vi "Compute Phasor Ratio References from UC Intersections.vi"(7 "mu+":dbl, 8 "error in (no error)":errorcluster, 9 "mu-":dbl, 10 "Phasor 1 (g, s)":T1, 11 "Phasor 2 (g, s)":T1) -> (0 "error out":errorcluster, 2 "Reference Phasor 2 (g, s)":T1, 3 "Reference Phasor 1 (g, s)":T1)   [LabVIEW 2021, in "Phasor.lvlib"]
uses:
  Phasor (g, s).ctl
  Phasor.lvlib
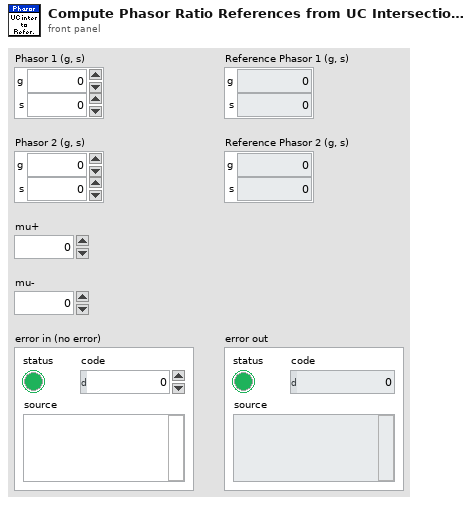
[diagram p1: front panel]
types:
  T1 = typedef "Phasor.lvlib/Phasor (g, s).ctl" = cluster{"g":dbl, "s":dbl}
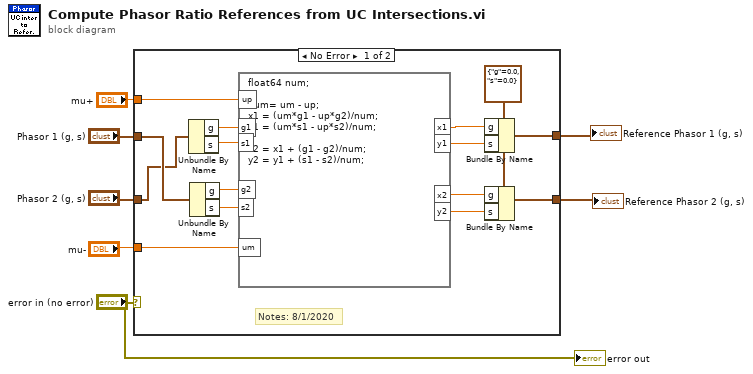
[diagram p0: block diagram]
diagram:
  n1 = case shown="No Error" "error in (no error)" {
    tunnel: "Phasor 1 (g, s)" -> [w9 w24]
    tunnel: "Phasor 2 (g, s)" -> [w8 w23]
    tunnel: "mu+" -> [w22 _]
    tunnel: "mu-" -> [w21 _]
    tunnel: [w14 w24] -> w3
    tunnel: [w10 w23] -> w2
    frame No Error {
      w13 = T1 {"g"=0.0, "s"=0.0} ("Reference Phasor 1 (g, s)")
      # "Notes: 8/1/2020"
      n2 = Unbundle By Name(w8) -> ("g"=w20:dbl, "s"=w19:dbl)
      n3 = Unbundle By Name(w9) -> ("g"=w18:dbl, "s"=w17:dbl)
      n4 = formula code="float64 num;\n\nnum= um - up;\nx1 = (um*g1 - up*g2)/num;\ny1 = (um*s1 - up*s2)/num;\n\nx2 = x1 + (g1 - g2)/num;\ny2 = y1 + (s1 - s2)/num;"("up"=w22, "um"=w21, "g1"=w20, "s1"=w19, "g2"=w18, "s2"=w17) -> ("x1"=w16:dbl, "y1"=w15:dbl, "x2"=w12:dbl, "y2"=w11:dbl)
      n5 = Bundle By Name(cluster=w13, "g"=w16, "s"=w15) -> (w14:T1)
      n6 = Bundle By Name(cluster=w13, "g"=w12, "s"=w11) -> (w10:T1)
    }
    frame Error {
    }
  }
  "Reference Phasor 2 (g, s)" <- w2
  "Reference Phasor 1 (g, s)" <- w3
  "error out" <- "error in (no error)"
